vi "CSM - Register Status Change.vi"(0 "CSM Name":string, 5 "Source CSM Name (* as Default)":string="*", 7 "Status":string, 9 "Response Message (if \"\", same as Source Message)":string, 11 "Error in":errorcluster caption="Error in (no error)") -> (4 "CSM Name(dup)":string, 15 "Error out":errorcluster)   [LabVIEW 2020, in "Communicable State Machine.lvlib"]
doc: "Register for notification of other CSM Module's status change. If \"Response Message\" is not connected or \"\" is the input, the same state name will be used for acting message.\n\n<b>Inputs:</b>\n - <b>CSM Name</b>: CSM Module name.\n - <b>Source CSM Name (* as Default)</b>: CSM who generates the status. You can use '*' for all modules generated the same <b>Status</b>\n - <b>Status</b>: The status string\n - <b>Response Message (if \"\", same as Source Message)</b>: After registered, If status change, this message will be received.\n - <b>Priority(T:As Status,F:As Interrupt)</b>: The Response Message will be inserted to the front of state queue if it's False, otherwise it wil be append to the tail.\n - <b>Error in</b>: Error cluster\n\n<b>Outputs:</b>\n - <b>CSM Name(dup)</b>: Return <b>CSM Name</b>\n - <b>Error out</b>: Error cluster"
uses:
  Communicable State Machine.lvlib
  Operation-BroadcastRegistry.ctl
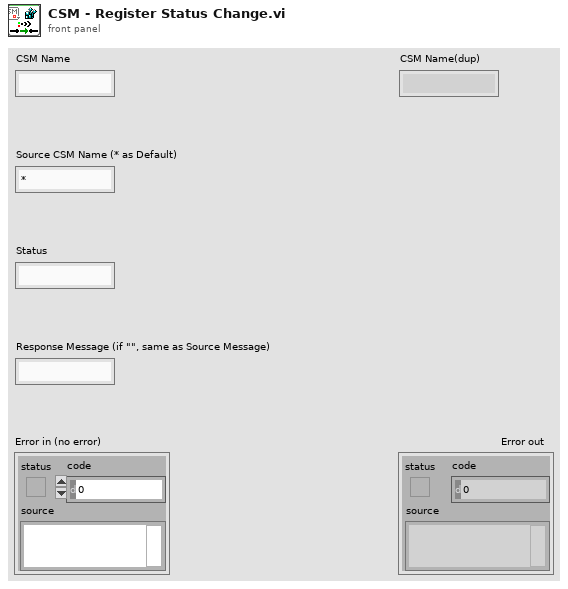
[diagram p1: front panel]
types:
  T1 = typedef "Communicable State Machine.lvlib/Operation-BroadcastRegistry.ctl" = enum16{"Delete Source Module", "Delete Target Module", "Remove Module", "Register", "Unregister", "Check", "List Status", "List Entries"}
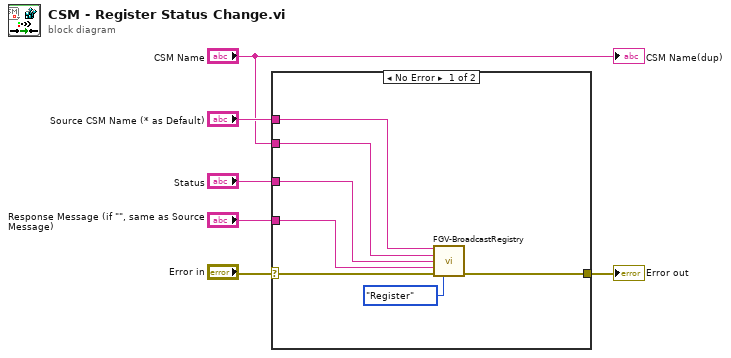
[diagram p0: block diagram]
diagram:
  n1 = case shown="No Error" "Error in" {
    selector: "Error in" -> [w12 w14]
    tunnel: [w11 w14] -> w5
    tunnel: "Response Message (if \"\", same as Source Message)" -> [w10 _]
    tunnel: "Status" -> [w9 _]
    tunnel: "CSM Name" -> [w8 _]
    tunnel: "Source CSM Name (* as Default)" -> [w7 _]
    frame No Error {
      n2 = call "FGV-BroadcastRegistry.vi"("Source"=w7, "Target"=w8, "Status"=w9, "API"=w10, "Error in"=w12, "Operation"=Operation-BroadcastRegistry."Register") -> ("Error out"=w11:errorcluster)  [unwired: 8 in, 1 out]
    }
    frame Error {
    }
  }
  "Error out" <- w5
  "CSM Name(dup)" <- "CSM Name"
